vi "日志报警状态存储 (子VI).vi"() -> ()   [LabVIEW 2016, in "斯坦道CODMn.lvlib"]
uses:
  <vilib>/ptbypt/NI_PtbyPt.lvlib
panel:
  out "多列列表框":i32(listbox)
  out "CODMn工作状态":T1(ring)
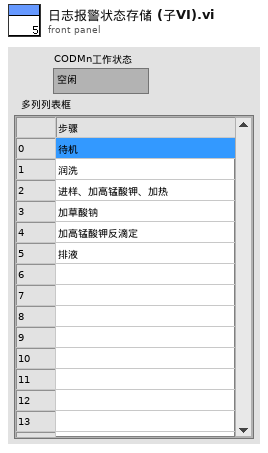
[diagram p1: front panel]
types:
  T1 = enum16{"空闲", "水样测试", "标样核查", "零点核查", "跨度核查", "空白测试", "平行样测试", "质控样", "空白校准", "标样校准", "加标回收"}
  T2 = typedef "报警信息字段定义.ctl" = cluster{"时间":timestamp, "参数":string, "报警信息":string, "备注":string, "code":u64, "platform_alarm_code":string}
  T3 = typedef "Alarm interface.lvlib/map in.ctl" = cluster{"name":string, "CN":string, "FirmwareVersion":string, "code":string}
  T4 = cluster{"时间标识":timestamp, "参数":string, "日志信息":string, "流程参数":string}
  T5 = cluster{"ORP故障":bool, "温控器故障":bool, "测量错误":bool, "校零错误":bool, "校标错误":bool, "进水样超量程":bool, "高锰酸钾报警":bool, "草酸钠报警":bool, "加热故障":bool, "缺硫酸告警":bool, "排液故障":bool, "缺水样告警":bool, "缺纯水或光值过低":bool, "缺标液告警":bool, "量程切换告警":bool, "滴定异常告警":bool, "光值过高告警":bool}
  T6 = cluster{"测量量程":dbl, "测量精度":dbl, "测量间隔":dbl, "消解温度":dbl, "消解时长":dbl, "空白校准时间":timestamp, "曲线截距":dbl, "曲线斜率":dbl, "测量检出限":dbl, "测量信号值":dbl, "线性相关系数":dbl, "二次多项式系数":dbl, "标样校准时间":timestamp, "稀释倍数":dbl, "三项式系数":dbl, "空白标定系数":dbl, "量程系数":dbl, "F0/ORPA":dbl, "F1/ORPB":dbl, "F2/ORPK":dbl, "F3":dbl, "F4":dbl, "F5":dbl, "F6":dbl, "F7":dbl, "X0/滴定数":dbl, "量程":dbl}
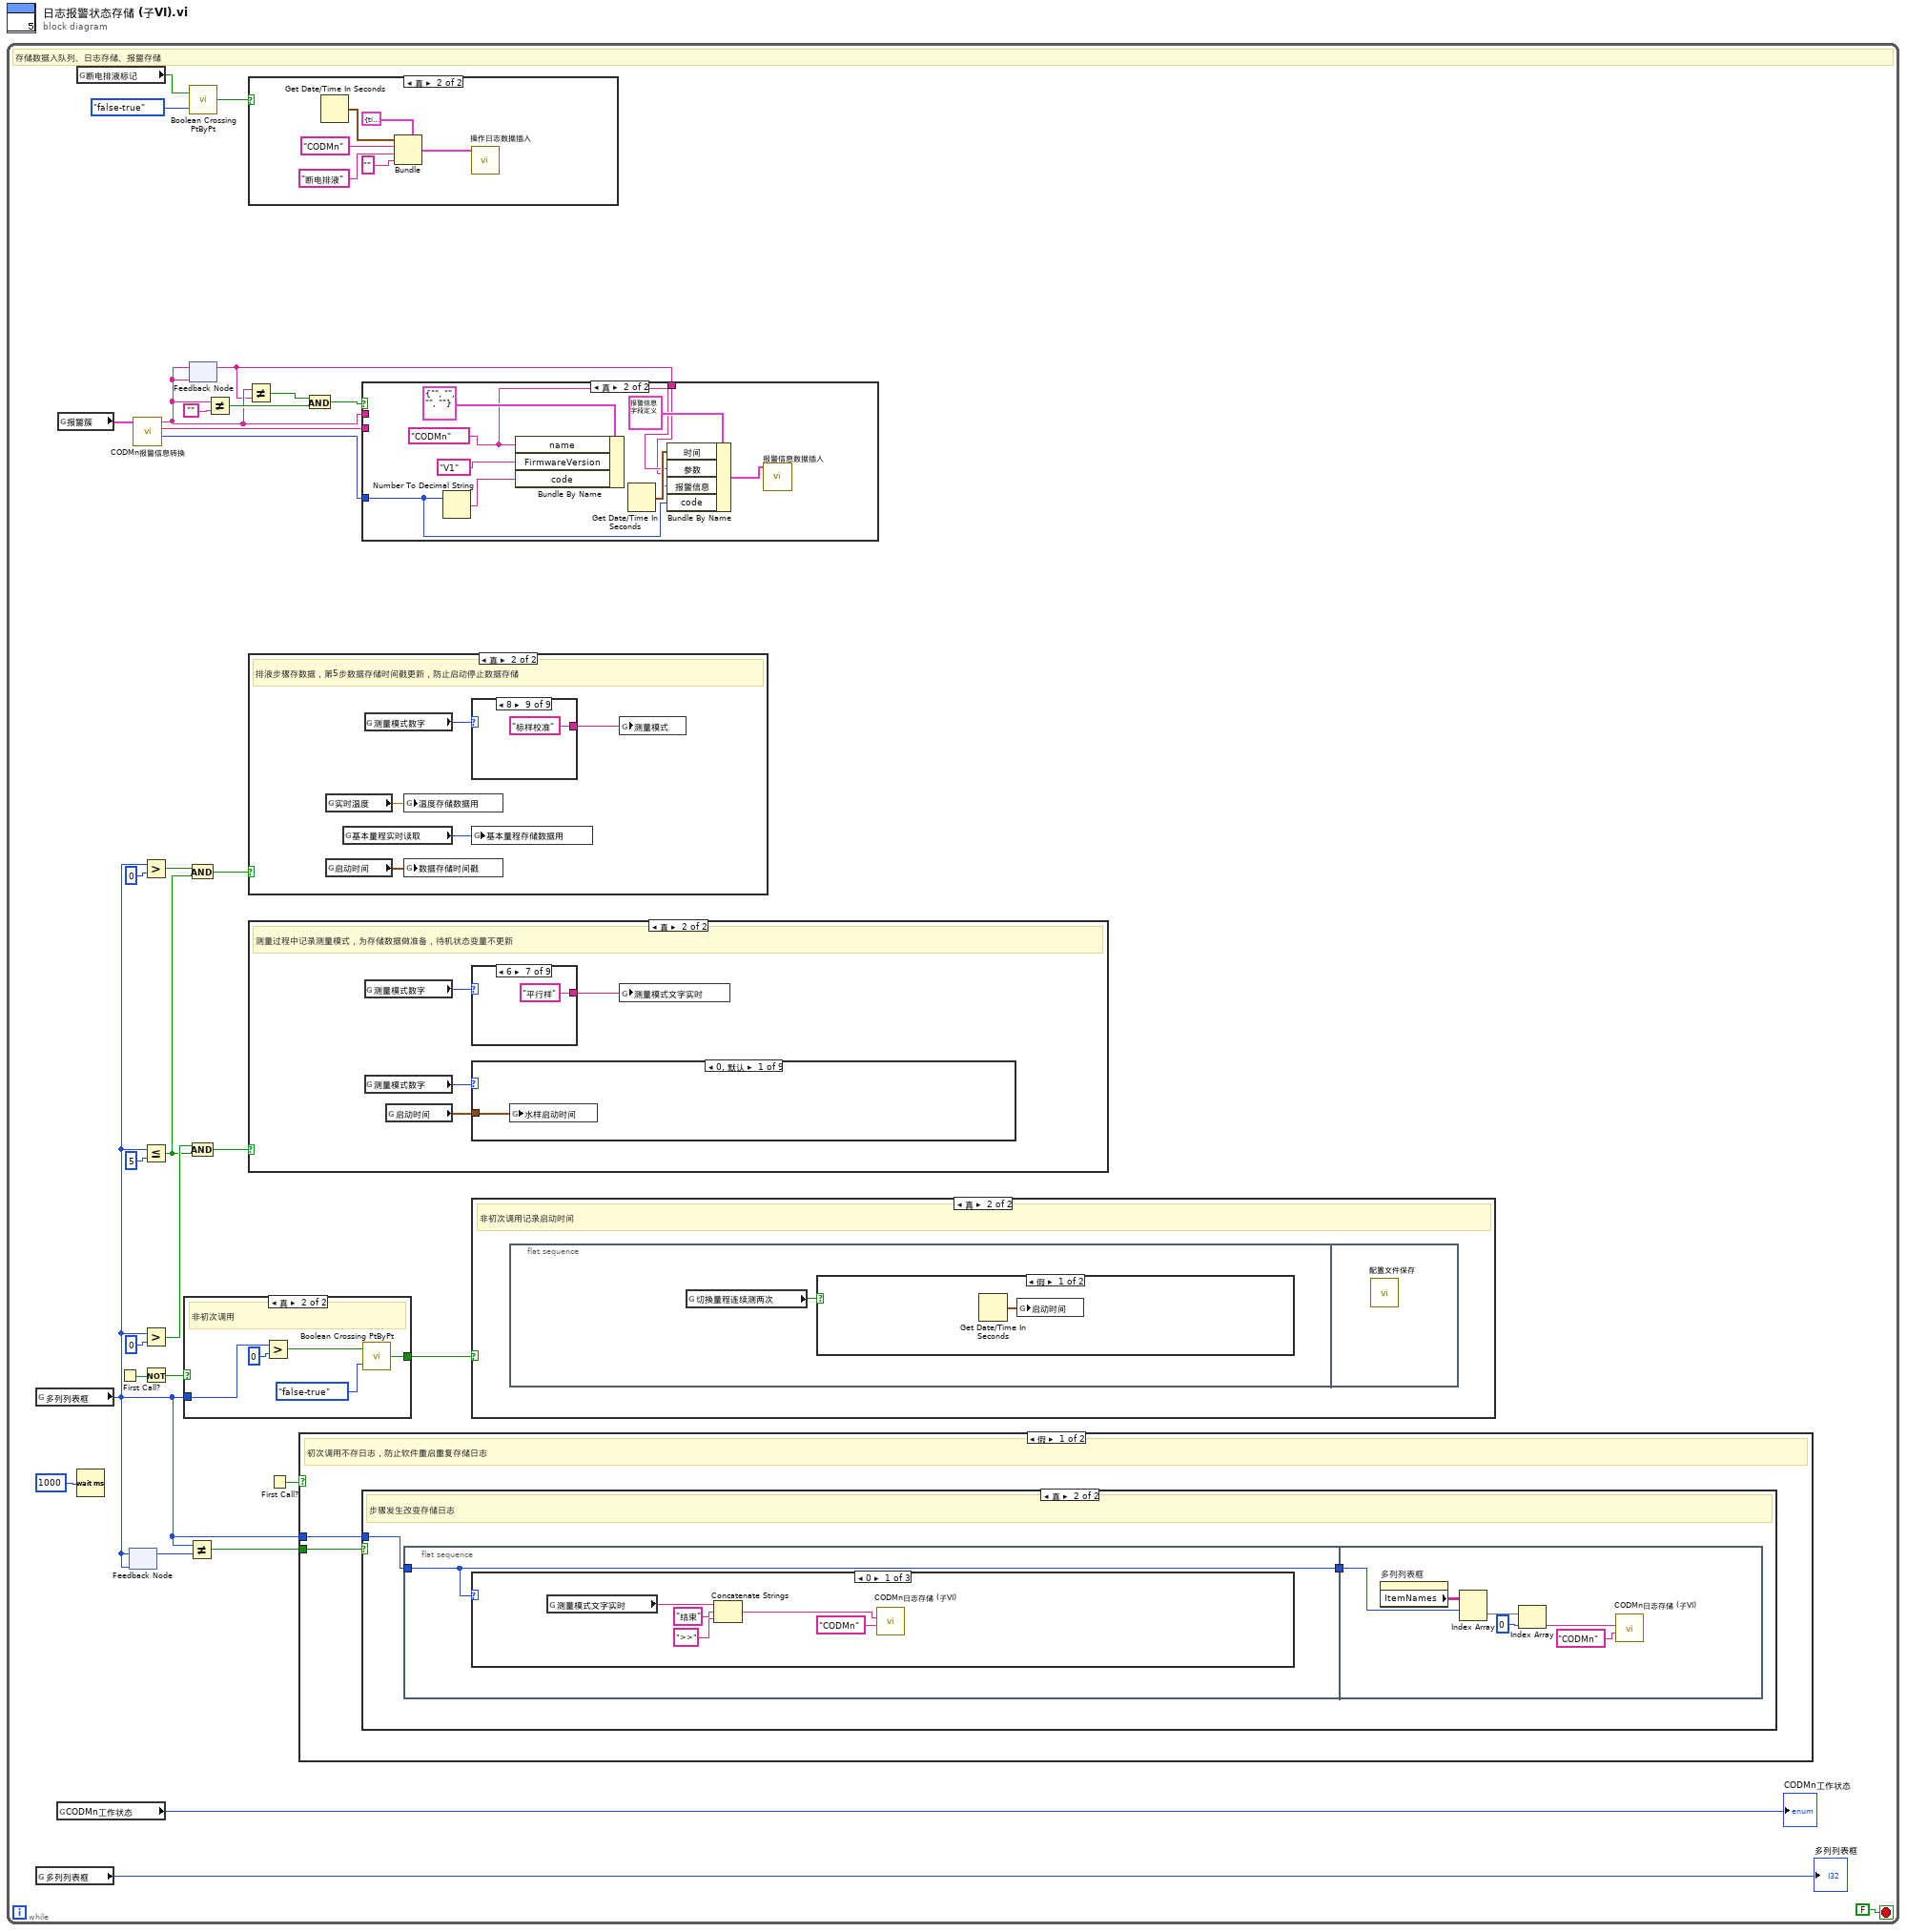
[diagram p0: block diagram]
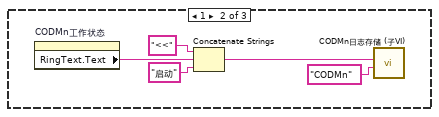
[diagram p3: hidden frame]
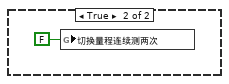
[diagram p10: hidden frame]
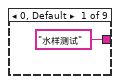
[diagram p12: hidden frame]
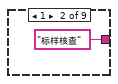
[diagram p13: hidden frame]
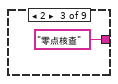
[diagram p14: hidden frame]
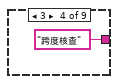
[diagram p15: hidden frame]
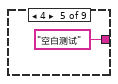
[diagram p16: hidden frame]
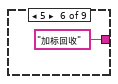
[diagram p17: hidden frame]
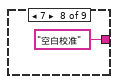
[diagram p18: hidden frame]
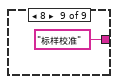
[diagram p19: hidden frame]
diagram:
  n1 = while {
    stop <- FALSE stop-if-true
    # "存储数据入队列、日志存储、报警存储"
    n2 = global read "运行时序全局变量.vi" "多列列表框"() -> (w6:i32)
    n3 = global read "运行时序全局变量.vi" "多列列表框"() -> (→"多列列表框":i32)
    n4 = global read "COD测量模式全局.vi" "CODMn工作状态"() -> (→"CODMn工作状态":T1)
    n5 = global read "COD内部交互全局.vi" "报警簇"() -> (w13:T5)
    n6 = global read "COD内部交互全局.vi" "断电排液标记"() -> (w12:bool)
    n7 = Wait (ms)(milliseconds to wait=u32 1000 ("等待时间（毫秒）")) -> ()  [unwired: 1 out]
    n8 = First Call?() -> (First Call?: T/F=w16:bool)
    n9 = feedback #1(w6) -> (w26:i32)
    n10 = feedback-in #1(w6) -> ()
    n11 = call "CODMn报警信息转换.vi"("报警簇"=w13) -> ("code"=w2:i32, "CODMN报警信息备注"=w3:string, "CODMN报警信息"=w17:string)  [unwired: 8 in]
    n12 = Greater?(x=w6, y=u16 0) -> (0:w8:bool)
    n13 = Less Or Equal?(x=w6, y=u16 5) -> (x <= y?=w7:bool)
    n14 = Greater?(x=w6, y=u16 0) -> (0:w31:bool)
    n15 = Not(x=w16) -> (.not. x?=w14:bool)
    n16 = case shown="真" w14 {
      selector: w14 -> [w53 _]
      tunnel: w6 -> [_ w55]
      tunnel: [w53 w54] -> w15
      frame False {
      }
      frame True {
        # "非初次调用"
        n17 = Greater?(x=w55, y=u16 0) -> (0:w58:bool)
        n18 = call <vilib>:"Boolean Crossing PtByPt.vi"("direction"=enum16{"either", "false-true", "true-false"}."false-true", "input"=w58) -> ("crossing"=w54:bool)  [unwired: 1 in]
      }
    }
    n19 = Not Equal?(x=w6, y=w26) -> (x != y?=w27:bool)
    n20 = And(x=w8, y=w7) -> (x .and. y?=w5:bool)
    n21 = And(x=w31, y=w7) -> (x .and. y?=w4:bool)
    n22 = call <vilib>:"Boolean Crossing PtByPt.vi"("direction"=enum16{"either", "false-true", "true-false"}."false-true", "input"=w12) -> ("crossing"=w22:bool)  [unwired: 1 in]
    n23 = feedback #2(w17) -> (w1:string)
    n24 = feedback-in #2(w17) -> ()
    n25 = Not Equal?(x=w17, y="") -> (x != y?=w21:bool)
    n26 = Not Equal?(x=w17, y=w1) -> (x != y?=w18:bool)
    n27 = case shown="真" w22 {
      frame False {
      }
      frame True {
        n28 = Get Date/Time In Seconds() -> (seconds since 1Jan1904=w73:timestamp)
        n29 = Bundle(cluster=T4 {"时间标识"=timestamp(0 s since 1904-01-01), "参数"="", "日志信息"="", "流程参数"=""} ("data in"), "时间标识"=w73, "参数"="CODMn" ("table输入"), "日志信息"="断电排液", "流程参数"="" ("table输入")) -> (w68:T4)
        n30 = call "操作日志数据插入.vi"("data"=w68) -> ()  [unwired: 9 in, 1 out]
      }
    }
    n31 = case shown="真" w5 {
      frame False {
      }
      frame True {
        # "排液步骤存数据，第5步数据存储时间戳更新，防止启动停止数据存储"
        n32 = global read "COD内部交互全局.vi" "实时温度"() -> (w101:dbl)
        n33 = global read "CODMn断电保存全局变量.vi" "启动时间"() -> (w102:timestamp)
        n34 = global read "COD内部交互全局.vi" "基本量程实时读取"() -> (w100:enum16{"L", "H", "AUTO"})
        n35 = global read "COD内部交互全局.vi" "测量模式数字"() -> (w99:i32)
        n36 = global write "COD内部交互全局.vi" "温度存储数据用"(w101) -> ()
        n37 = global write "COD内部交互全局.vi" "数据存储时间戳"(w102) -> ()
        n38 = case shown="8" w99 {
          tunnel: ["水样测试" ("测量模式") "标样核查" ("测量模式") "零点核查" ("测量模式") "跨度核查" ("测量模式") "空白测试" ("测量模式") "加标回收" ("测量模式") "平行样" ("测量模式") "空白校准" ("测量模式") "标样校准" ("测量模式")] -> w98
          frame 0, Default {
          }
          frame 1 {
          }
          frame 2 {
          }
          frame 3 {
          }
          frame 4 {
          }
          frame 5 {
          }
          frame 6 {
          }
          frame 7 {
          }
          frame 8 {
          }
        }
        n39 = global write "COD内部交互全局.vi" "基本量程存储数据用"(w100) -> ()
        n40 = global write "CODMn断电保存全局变量.vi" "测量模式"(w98) -> ()
      }
    }
    n41 = case shown="真" w4 {
      frame False {
      }
      frame True {
        # "测量过程中记录测量模式，为存储数据做准备，待机状态变量不更新"
        n42 = global read "COD内部交互全局.vi" "测量模式数字"() -> (w77:i32)
        n43 = global read "COD内部交互全局.vi" "测量模式数字"() -> (w79:i32)
        n44 = global read "CODMn断电保存全局变量.vi" "启动时间"() -> (w80:timestamp)
        n45 = case shown="6" w77 {
          tunnel: ["水样测试" ("测量模式") "标样核查" ("测量模式") "零点核查" ("测量模式") "跨度核查" ("测量模式") "空白测试" ("测量模式") "加标回收" ("测量模式") "平行样" ("测量模式") "空白校准" ("测量模式") "标样校准" ("测量模式")] -> w78
          frame 0, Default {
          }
          frame 1 {
          }
          frame 2 {
          }
          frame 3 {
          }
          frame 4 {
          }
          frame 5 {
          }
          frame 6 {
          }
          frame 7 {
          }
          frame 8 {
          }
        }
        n46 = case shown="0, 默认" w79 {
          tunnel: w80 -> [w90 _ _ _ _ w91 _ w92 w95]
          frame 0, Default {
            n47 = global write "COD测量模式全局.vi" "水样启动时间"(w90) -> ()
          }
          frame 1 {
          }
          frame 2 {
          }
          frame 3 {
          }
          frame 4 {
          }
          frame 5 {
            n48 = global write "COD测量模式全局.vi" "加标回收启动时间"(w91) -> ()
          }
          frame 6 {
          }
          frame 7 {
            n49 = global read "CODMn断电保存全局变量.vi" "CODMn仪器参数"() -> (w94:T6)
            n50 = Bundle By Name(cluster=w94, "空白校准时间"=w92) -> (w93:T6)
            n51 = global write "CODMn断电保存全局变量.vi" "CODMn仪器参数"(w93) -> ()
          }
          frame 8 {
            n52 = global read "CODMn断电保存全局变量.vi" "CODMn仪器参数"() -> (w97:T6)
            n53 = Bundle By Name(cluster=w97, "标样校准时间"=w95) -> (w96:T6)
            n54 = global write "CODMn断电保存全局变量.vi" "CODMn仪器参数"(w96) -> ()
          }
        }
        n55 = global write "COD测量模式全局.vi" "测量模式文字实时"(w78) -> ()
      }
    }
    n56 = First Call?() -> (First Call?: T/F=w28:bool)
    n57 = case shown="假" w28 {
      tunnel: w27 -> [w33 _]
      tunnel: w6 -> [w32 _]
      frame False {
        # "初次调用不存日志，防止软件重启重复存储日志"
        n58 = case shown="真" w33 {
          tunnel: w32 -> [_ w35]
          frame False {
          }
          frame True {
            # "步骤发生改变存储日志"
            n59 = flat-sequence {
              tunnel: w35 -> [w36]
              tunnel: [w36] -> w34
              tunnel: w34 -> [w52]
              frame #0 {
                n60 = case shown="0" w36 {
                  frame 0 {
                    n61 = global read "COD测量模式全局.vi" "测量模式文字实时"() -> (w38:string)
                    n62 = Concatenate Strings(w38, "结束" ("字符串"), ">>") -> (w41:string)
                    n63 = call "CODMn日志存储 (子VI).vi"("参数"="CODMn" ("table输入"), "日志信息"=w41) -> ()  [unwired: 10 in]
                  }
                  frame 1 {
                    n64 = property on="CODMn工作状态" class="Enum (严格)"() -> ("RingText.Text"=w42:string)  [unwired: 2 in, 2 out]
                    n65 = Concatenate Strings("<<", w42, "启动" ("字符串")) -> (w43:string)
                    n66 = call "CODMn日志存储 (子VI).vi"("参数"="CODMn" ("table输入"), "日志信息"=w43) -> ()  [unwired: 10 in]
                  }
                  frame 2, Default {
                  }
                }
              }
              frame #1 {
                n67 = property on="多列列表框" class="MCListbox (严格)"() -> ("ItemNames"=w47:string[][])  [unwired: 2 in, 2 out]
                n68 = Index Array(array=w47, index (row)=w52) -> (element=w50:string[])  [unwired: 1 in]
                n69 = Index Array(array=w50, index=0 ("索引")) -> (element=w48:string)
                n70 = call "CODMn日志存储 (子VI).vi"("参数"="CODMn" ("table输入"), "日志信息"=w48) -> ()  [unwired: 10 in]
              }
            }
          }
        }
      }
      frame True {
      }
    }
    n71 = And(x=w18, y=w21) -> (x .and. y?=w19:bool)
    n72 = case shown="真" w19 {
      tunnel: w17 -> [_ _]
      tunnel: w3 -> [_ _]
      tunnel: w2 -> [_ w60]
      tunnel: w1 -> [_ w61]
      frame False {
      }
      frame True {
        w62 = "CODMn" ("componentParent")
        n73 = Number To Decimal String(number=w60) -> (decimal integer string=w66:string)  [unwired: 1 in]
        n74 = Bundle By Name(cluster=T3 {"name"="", "CN"="", "FirmwareVersion"="", "code"=""} ("map in"), "name"=w62, "FirmwareVersion"="V1" ("ver"), "code"=w66) -> ()  [unwired: 1 out]
        n75 = Get Date/Time In Seconds() -> (seconds since 1Jan1904=w63:timestamp)
        n76 = Bundle By Name(cluster=T2 {"时间"=timestamp(0 s since 1904-01-01), "参数"="", "报警信息"="", "备注"="", "code"=0, "platform_alarm_code"=""} ("data"), "时间"=w63, "参数"=w62, "报警信息"=w61, "code"=w60) -> (w59:T2)
        n77 = call "报警信息数据插入.vi"("data"=w59) -> ()  [unwired: 9 in, 1 out]
      }
    }
    n78 = case shown="真" w15 {
      frame False {
      }
      frame True {
        # "非初次调用记录启动时间"
        n79 = flat-sequence {
          frame #0 {
            n80 = global read "COD内部交互全局.vi" "切换量程连续测两次"() -> (w74:bool)
            n81 = case shown="假" w74 {
              frame False {
                n82 = Get Date/Time In Seconds() -> (seconds since 1Jan1904=w75:timestamp)
                n83 = global write "CODMn断电保存全局变量.vi" "启动时间"(w75) -> ()
              }
              frame True {
                n84 = global write "COD内部交互全局.vi" "切换量程连续测两次"(FALSE ("切换量程连续测两次")) -> ()
              }
            }
          }
          frame #1 {
            n85 = call "配置文件保存.vi"() -> ()  [unwired: 12 in]
          }
        }
      }
    }
  }
